vi "mhk_integration_differentiation.vi"() -> ()   [LabVIEW 2011]
uses:
  <vilib>/Analysis/2dsp.llb/Integral Method.ctl
  <vilib>/Analysis/8numeric.llb/1D Numeric Integration.vi
  <vilib>/Analysis/NI_AALPro.lvlib
panel:
  out "delta x":dbl=0.05
  in  "derivative method":u16(ring) items=["2nd Order Central", "4th Order Central", "Forward", "Backward"]
  out "dX/dt":dbl[](array[numeric])=[-15.405227750880535, -30.395841112644344, -28.145520160101633, -23.054920593250632, -15.276733071401564, -5.271698036249486, 6.188174004936413, 18.054279002520012, 29.07824972451194, 37.93026851589308, 43.351980328637985, 44.33025322000254, 40.27144040968473, 31.150672305651614, 17.608356258271485, 0.9677054074756342, -16.84637570596834, -33.49511954970159, -46.51247148805192, -53.663686312401836, -53.33049811465331, -44.86232062329084, -28.825388704008706, -7.085296642689287, 17.324694833852234, 40.56679586212218, 58.569289985031865, 67.7344902418929, 65.67143929398677, 51.812044837809175, 27.76429029534297, -2.7181408474015356, -34.21220877857431, -60.524775844542695, -75.89257709186059, -76.26820840833531, -60.41567294723322, -30.530555876497694, 7.840573916741711, 46.6786745205185, 32.548804828616404]
  out "function vector":dbl[](array[numeric])=[2.8782945992814364, 1.337771824193383, -0.16128951198299823, -1.4767801918167804, -2.4667815713080614, -3.004453498956937, -2.99395137493301, -2.3856360984632956, -1.1885234746810087, 0.5221888739878988, 2.6045033769083, 4.857386906851698, 7.037528698908554, 8.88453094782017, 10.152595929473716, 10.645366573647319, 10.249366470221279, 8.960729003050485, 6.8998545152511195, 4.309481854245292, 1.5334858840109358, -1.0235679572200391, -2.9527461783181486, -3.90610682762091, -3.6612758425870773, -2.1736373442356864, 0.3954037436251405, 3.6832916542675007, 7.168852767814431, 10.250435583666178, 12.350057251595349, 13.026864613200475, 12.078243166855195, 9.605643735343044, 6.0257655824009255, 2.0163860261569853, -1.6010552584326065, -4.025181268566337, -4.654110846082376, -3.241123876892166, 0.013756605969474478]
  out "accumulated da vector":dbl[](array[numeric])=[0.0, 0.10540166058687049, 0.1348137183921301, 0.09386197579713564, -0.004727068280985416, -0.14150794503761038, -0.29146806688485905, -0.42595775371976674, -0.5153117430483743, -0.5319701080657021, -0.45380280179329713, -0.2672555446992972, 0.03011734544470912, 0.42816883661292726, 0.9040970085452744, 1.4240460711233003, 1.9464143972200154, 2.4266667840518097, 2.82318137200935, 3.10341478124676, 3.2494889747031657, 3.262236922872938, 3.1628290694844834, 2.991357744336007, 2.802173177580807, 2.6563003479102383, 2.6118445078949746, 2.7138118928422905, 2.9851155033943386, 3.4205977121813538, 3.985610033062892, 4.620033079682788, 5.24766077418418, 5.789757946739136, 6.180543179682735, 6.381596969896682, 6.391980239089792, 6.251324325914818, 6.0343420230486, 5.836961154974237, 5.756276973201169]
  out "Integral X":dbl[](array[numeric])=[0.0, 0.10540166058687049, 0.1348137183921301, 0.09386197579713564, -0.004727068280985416, -0.14150794503761038, -0.29146806688485905, -0.4259577537197667, -0.5153117430483743, -0.5319701080657021, -0.45380280179329713, -0.2672555446992972, 0.030117345444709127, 0.42816883661292726, 0.9040970085452744, 1.4240460711233003, 1.9464143972200152, 2.4266667840518092, 2.8231813720093495, 3.1034147812467596, 3.2494889747031652, 3.2622369228729378, 3.162829069484483, 2.9913577443360064, 2.8021731775808068, 2.656300347910238, 2.611844507894974, 2.71381189284229, 2.985115503394338, 3.4205977121813533, 3.9856100330628914, 4.620033079682787, 5.247660774184179, 5.789757946739135, 6.180543179682735, 6.381596969896682, 6.391980239089792, 6.251324325914818, 6.0343420230486, 5.836961154974237, 5.756276973201169]
  out "raw da vector":dbl[](array[numeric])=[0.0, 0.10540166058687049, 0.029412057805259618, -0.04095174259499447, -0.09858904407812105, -0.13678087675662495, -0.1499601218472487, -0.13448968683490767, -0.08935398932860761, -0.016658365017327748, 0.07816730627240498, 0.18654725709399994, 0.2973728901440063, 0.39805149116821814, 0.47592817193234715, 0.5199490625780259, 0.522368326096715, 0.4802523868317941, 0.39651458795754013, 0.2802334092374103, 0.14607419345640568, 0.012747948169772417, -0.0994078533884547, -0.1714713251484765, -0.18918456675519968, -0.1458728296705691, -0.04445584001526365, 0.10196738494731604, 0.27130361055204827, 0.43548220878701527, 0.5650123208815382, 0.6344230466198957, 0.6276276945013918, 0.542097172554956, 0.39078523294359924, 0.20105379021394776, 0.010383269193109468, -0.14065591317497358, -0.21698230286621786, -0.19738086807436356, -0.0806841817730673]
  out "function\nvector\nsize":i32=41
  out "da\nvector\nsize":i32=41
  out "1D integration\nresult":dbl=5.75627697320117 format="%0.5f"
  out "Running Integral Graph":cluster{"Lower limit \"a\"":dbl, dbl, dbl[][]}(graph)={"Lower limit \"a\""=2.8, 0.05, [[0.0, 0.10540166058687049, 0.029412057805259618, -0.04095174259499447, -0.09858904407812105, -0.13678087675662495, -0.1499601218472487, -0.13448968683490767, -0.08935398932860761, -0.016658365017327748, 0.07816730627240498, 0.18654725709399994, 0.2973728901440063, 0.39805149116821814, 0.47592817193234715, 0.5199490625780259, 0.522368326096715, 0.4802523868317941, 0.39651458795754013, 0.2802334092374103, 0.14607419345640568, 0.012747948169772417, -0.0994078533884547, -0.1714713251484765, -0.18918456675519968, -0.1458728296705691, -0.04445584001526365, 0.10196738494731604, 0.27130361055204827, 0.43548220878701527, 0.5650123208815382, 0.6344230466198957, 0.6276276945013918, 0.542097172554956, 0.39078523294359924, 0.20105379021394776, 0.010383269193109468, -0.14065591317497358, -0.21698230286621786, -0.19738086807436356, -0.0806841817730673], [0.0, 0.10540166058687049, 0.1348137183921301, 0.09386197579713564, -0.004727068280985416, -0.14150794503761038, -0.29146806688485905, -0.42595775371976674, -0.5153117430483743, -0.5319701080657021, -0.45380280179329713, -0.2672555446992972, 0.03011734544470912, 0.42816883661292726, 0.9040970085452744, 1.4240460711233003, 1.9464143972200154, 2.4266667840518097, 2.82318137200935, 3.10341478124676, 3.2494889747031657, 3.262236922872938, 3.1628290694844834, 2.991357744336007, 2.802173177580807, 2.6563003479102383, 2.6118445078949746, 2.7138118928422905, 2.9851155033943386, 3.4205977121813538, 3.985610033062892, 4.620033079682788, 5.24766077418418, 5.789757946739136, 6.180543179682735, 6.381596969896682, 6.391980239089792, 6.251324325914818, 6.0343420230486, 5.836961154974237, 5.756276973201169], [0.0, 0.10540166058687049, 0.1348137183921301, 0.09386197579713564, -0.004727068280985416, -0.14150794503761038, -0.29146806688485905, -0.4259577537197667, -0.5153117430483743, -0.5319701080657021, -0.45380280179329713, -0.2672555446992972, 0.030117345444709127, 0.42816883661292726, 0.9040970085452744, 1.4240460711233003, 1.9464143972200152, 2.4266667840518092, 2.8231813720093495, 3.1034147812467596, 3.2494889747031652, 3.2622369228729378, 3.162829069484483, 2.9913577443360064, 2.8021731775808068, 2.656300347910238, 2.611844507894974, 2.71381189284229, 2.985115503394338, 3.4205977121813533, 3.9856100330628914, 4.620033079682787, 5.247660774184179, 5.789757946739135, 6.180543179682735, 6.381596969896682, 6.391980239089792, 6.251324325914818, 6.0343420230486, 5.836961154974237, 5.756276973201169]]}
  in  "Plot BG Color":bool
  out "Approx. Integral \nover entire range\ndone incrementally":dbl=5.75627697320117
  out "Approx. Integral \nover entire range\ndone en masse":dbl=5.75627697320117
  out "Function Graph":cluster{"Lower limit \"a\"":dbl, dbl, dbl[][]}(graph)={"Lower limit \"a\""=2.8, 0.05, [[2.8782945992814364, 1.337771824193383, -0.16128951198299823, -1.4767801918167804, -2.4667815713080614, -3.004453498956937, -2.99395137493301, -2.3856360984632956, -1.1885234746810087, 0.5221888739878988, 2.6045033769083, 4.857386906851698, 7.037528698908554, 8.88453094782017, 10.152595929473716, 10.645366573647319, 10.249366470221279, 8.960729003050485, 6.8998545152511195, 4.309481854245292, 1.5334858840109358, -1.0235679572200391, -2.9527461783181486, -3.90610682762091, -3.6612758425870773, -2.1736373442356864, 0.3954037436251405, 3.6832916542675007, 7.168852767814431, 10.250435583666178, 12.350057251595349, 13.026864613200475, 12.078243166855195, 9.605643735343044, 6.0257655824009255, 2.0163860261569853, -1.6010552584326065, -4.025181268566337, -4.654110846082376, -3.241123876892166, 0.013756605969474478], [-15.405227750880535, -30.395841112644344, -28.145520160101633, -23.054920593250632, -15.276733071401564, -5.271698036249486, 6.188174004936413, 18.054279002520012, 29.07824972451194, 37.93026851589308, 43.351980328637985, 44.33025322000254, 40.27144040968473, 31.150672305651614, 17.608356258271485, 0.9677054074756342, -16.84637570596834, -33.49511954970159, -46.51247148805192, -53.663686312401836, -53.33049811465331, -44.86232062329084, -28.825388704008706, -7.085296642689287, 17.324694833852234, 40.56679586212218, 58.569289985031865, 67.7344902418929, 65.67143929398677, 51.812044837809175, 27.76429029534297, -2.7181408474015356, -34.21220877857431, -60.524775844542695, -75.89257709186059, -76.26820840833531, -60.41567294723322, -30.530555876497694, 7.840573916741711, 46.6786745205185, 32.548804828616404]]}
  in  "Divisions \"N\"":dbl=40.0
  in  "Upper limit \"b\"":dbl=4.8
  in  "Lower limit \"a\"":dbl=2.8
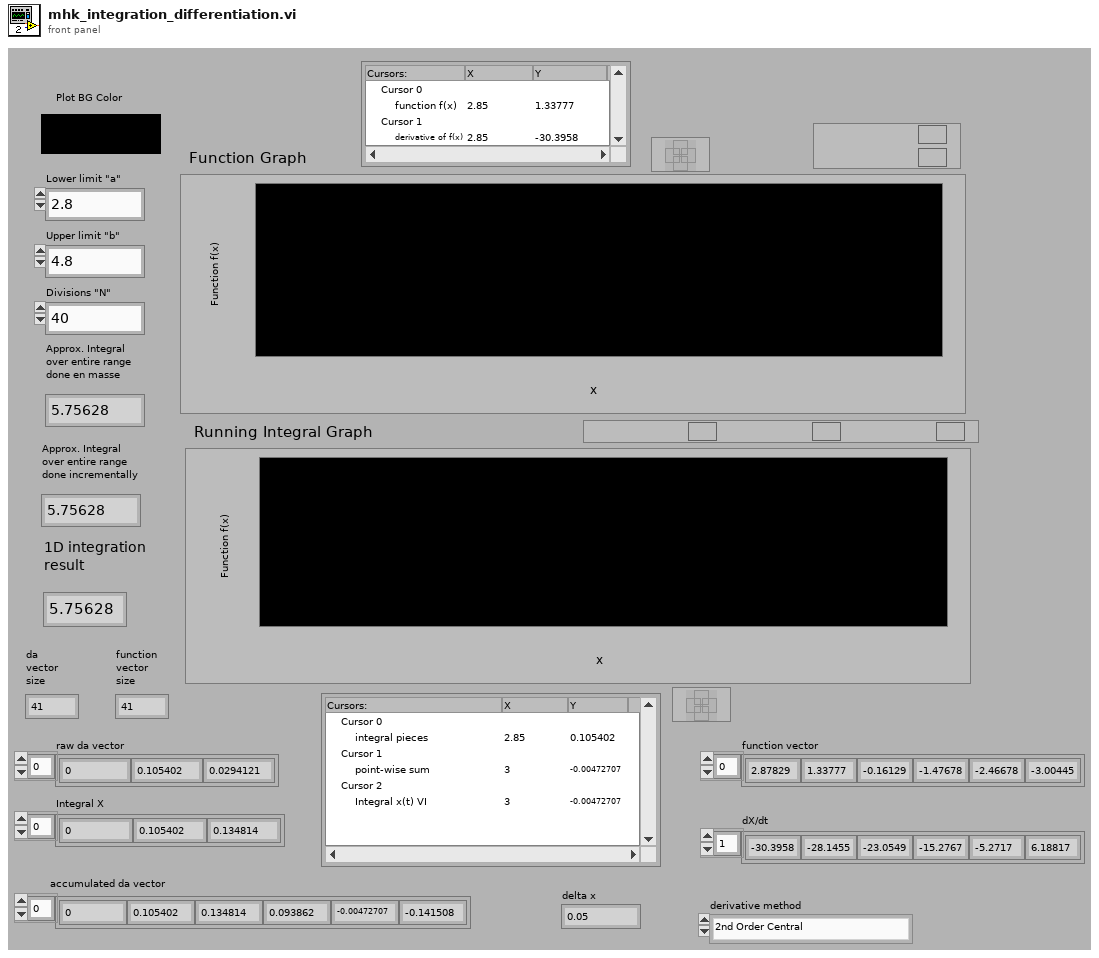
[diagram p1: front panel]
types:
  T1 = typedef "NI_AALPro.lvlib/Integral Method.ctl" = i32
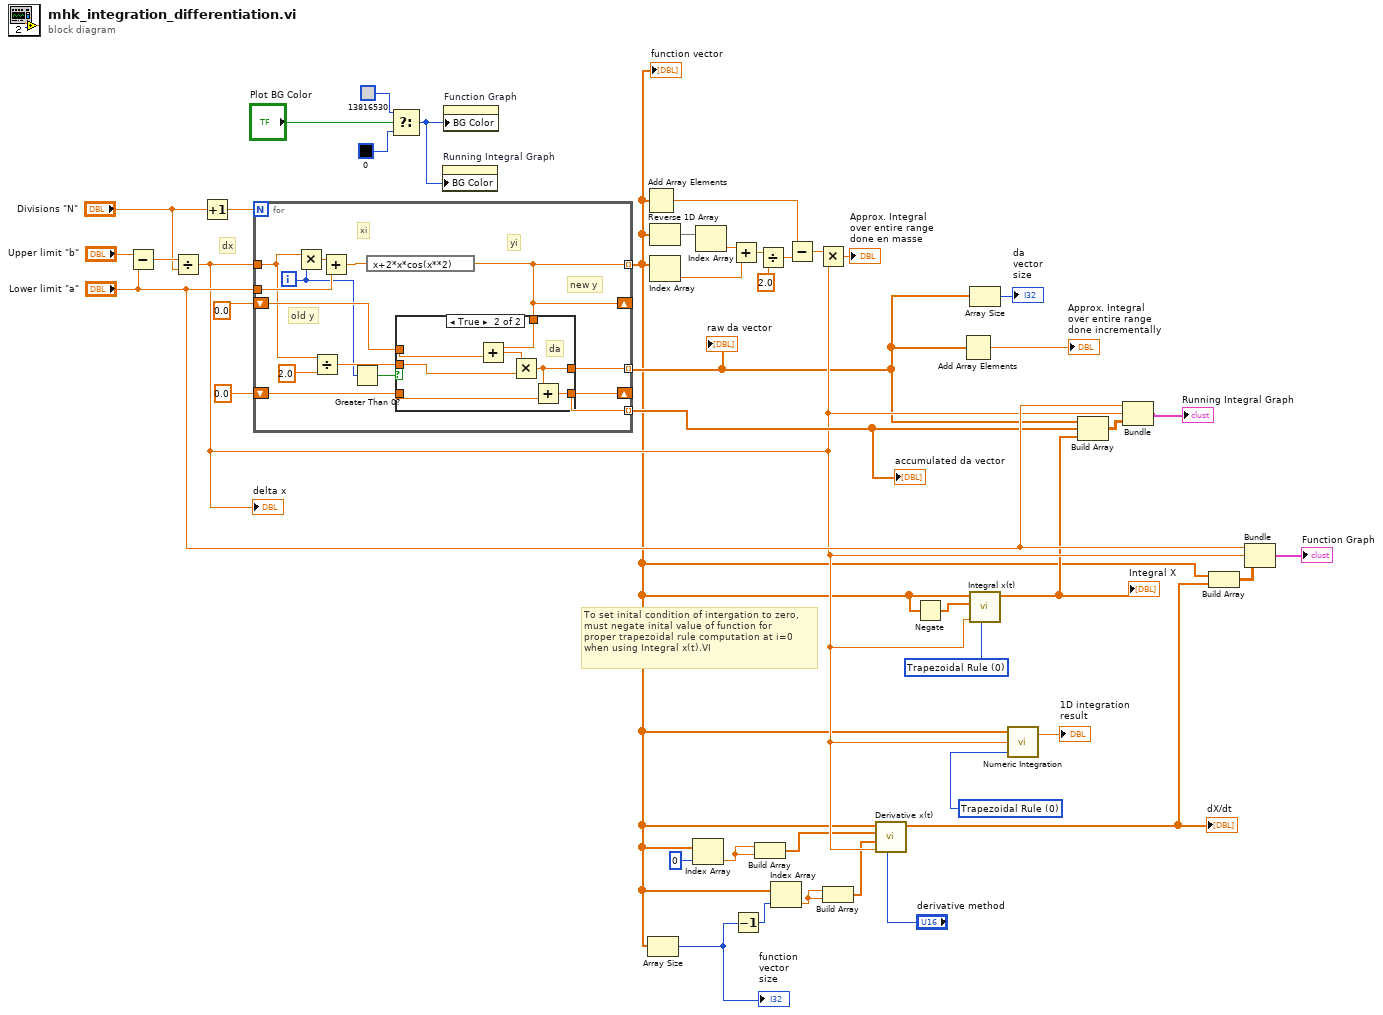
[diagram p0: block diagram]
diagram:
  w20 = T1 0 items=["Trapezoidal Rule", "Simpson's Rule", "Simpson's 3/8 Rule", "Bode Rule"] ("integration method")
  w22 = T1 0 items=["Trapezoidal Rule", "Simpson's Rule", "Simpson's 3/8 Rule", "Bode Rule"] ("integration method")
  # "To set inital condition of intergation to zero,\nmust negate inital value of function for \nproper trapezoidal rule computation at i=0 \nwhen using Integral x(t).VI"
  # "dx"
  n1 = Subtract(x="Upper limit \"b\"", y="Lower limit \"a\"") -> (x-y=w43:dbl)
  n2 = Divide(x=w43, y="Divisions \"N\"") -> (x/y=w19:dbl)
  "delta x" <- w19
  n3 = Increment(x="Divisions \"N\"") -> (x+1=w42:dbl)
  n4 = for {
    N: w42 -> [_]
    tunnel: w19 -> [w46]
    tunnel: "Lower limit \"a\"" -> [w56]
    tunnel: [w54] -> w3 mode=indexing
    shift-right: [w54] -> _
    shift-left: 0.0 -> [w53]
    tunnel: [w50] -> w13 mode=indexing
    shift-right: [w48] -> _
    shift-left: 0.0 -> [w49]
    tunnel: [w48] -> w24 mode=indexing
    i -> [w45]
    # "new y"
    # "old y"
    # "yi"
    # "xi"
    n5 = Multiply(x=w46, y=w45) -> (x*y=w57:dbl)
    n6 = Divide(x=w46, y=2.0) -> (x/y=w51:dbl)
    n7 = Add(x=w57, y=w56) -> (x+y=w55:dbl)
    n8 = Greater Than 0?(x=w45) -> (x > 0?=w47:bool)
    n9 = expression code="x+2*x*cos(x**2)"(w55) -> (w54:dbl)
    n10 = case shown="True" w47 {
      tunnel: w54 -> [_ w65]
      tunnel: w53 -> [_ w64]
      tunnel: w51 -> [_ w62]
      tunnel: [w58 w61] -> w50
      tunnel: w49 -> [w58 w60]
      tunnel: [w58 w59] -> w48
      frame False {
      }
      frame True {
        # "da"
        n11 = Add(x=w65, y=w64) -> (x+y=w63:dbl)
        n12 = Multiply(x=w63, y=w62) -> (x*y=w61:dbl)
        n13 = Add(x=w61, y=w60) -> (x+y=w59:dbl)
      }
    }
  }
  "raw da vector" <- w13
  "accumulated da vector" <- w24
  "function vector" <- w3
  n14 = Select(t=u32 13816530, s="Plot BG Color", f=u32 0) -> (s? t:f=w25:u32)
  n15 = property on="Running Integral Graph" class="WFGraph (strict)"("BG Color"=w25) -> ()  [unwired: 2 in, 2 out]
  n16 = property on="Function Graph" class="WFGraph (strict)"("BG Color"=w25) -> ()  [unwired: 2 in, 2 out]
  n17 = Add Array Elements(numeric array=w3) -> (sum=w34:dbl)
  n18 = Array Size(array=w3) -> (size(s)=w7:i32)
  "function\nvector\nsize" <- w7
  n19 = Reverse 1D Array(array=w3) -> (reversed array=w40:dbl[])
  n20 = Index Array(array=w3) -> (element=w38:dbl)  [unwired: 1 in]
  n21 = Index Array(array=w3, index=0) -> (element=w9:dbl)
  n22 = Index Array(array=w40) -> (element=w39:dbl)  [unwired: 1 in]
  n23 = Add(x=w39, y=w38) -> (x+y=w37:dbl)
  n24 = Decrement(x=w7) -> (x-1=w6:i32)
  n25 = Build Array(w9, w9) -> (w8:dbl[])
  n26 = Divide(x=w37, y=2.0) -> (x/y=w35:dbl)
  n27 = Index Array(array=w3, index=w6) -> (element=w5:dbl)
  n28 = Subtract(x=w34, y=w35) -> (x-y=w33:dbl)
  n29 = Multiply(x=w33, y=w19) -> (x*y=→"Approx. Integral \nover entire range\ndone en masse":dbl)
  n30 = Build Array(w5, w5) -> (w4:dbl[])
  n31 = call <vilib>:"Derivative x(t).vi"("method"="derivative method", "dt"=w19, "Final Condition"=w4, "Initial Condition"=w8, "X"=w3) -> ("dX/dt"=w2:dbl[])  [unwired: 5 in, 1 out]
  "dX/dt" <- w2
  n32 = Negate(x=w3) -> (-x=w12:dbl[])
  n33 = Add Array Elements(numeric array=w13) -> (sum=→"Approx. Integral \nover entire range\ndone incrementally":dbl)
  n34 = Array Size(array=w13) -> (size(s)=→"da\nvector\nsize":i32)
  n35 = call <vilib>:"Integral x(t).vi"("integration method"=w20, "dt"=w19, "Initial Condition"=w12, "X"=w3) -> ("Integral X"=w15:dbl[])  [unwired: 6 in, 1 out]
  "Integral X" <- w15
  n36 = call-poly <vilib>:"Numeric Integration.vi"("integration method"=w22, "dt"=w19, "Input Array"=w3) -> ("result"=→"1D integration\nresult":dbl)  [unwired: 1 out]
  n37 = Build Array(w13, w24, w15) -> (w23:dbl[][])
  n38 = Bundle("Lower limit \"a\""="Lower limit \"a\"", w19, w23) -> (→"Running Integral Graph":cluster{"Lower limit \"a\"":dbl, dbl, dbl[][]})  [unwired: 1 in]
  n39 = Build Array(w3, w2) -> (w1:dbl[][])
  n40 = Bundle("Lower limit \"a\""="Lower limit \"a\"", w19, w1) -> (→"Function Graph":cluster{"Lower limit \"a\"":dbl, dbl, dbl[][]})  [unwired: 1 in]
